vi "Write DIO Threshold.vi"(7 "Logic Threshold (%)":dbl, 8 "error in (no error)":errorcluster, 9 "Chip Address (A2 A1 A0)":T2 max=7, 10 "Slot #":T1 max=15, 11 "Rack #":u8) -> (0 "error out":errorcluster, 3 "FIFO SPI Message":u64 format="%b")   [LabVIEW 2014, in "SLSC configuration Shared.lvlib"]
uses:
  SLSC configuration Shared.lvlib
  MCP23S17/Chip Address.ctl
  SPI Utility/Slot #.ctl
  MCP23S17/IOCON BANK 0 Reg Addresses.ctl
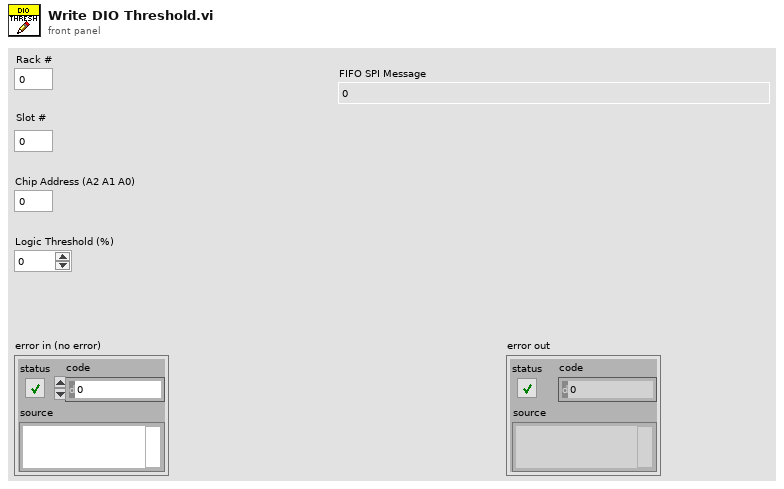
[diagram p1: front panel]
types:
  T1 = typedef "SLSC configuration Shared.lvlib/Slot #.ctl" = u8
  T2 = typedef "SLSC configuration Shared.lvlib/Chip Address.ctl" = u8
  T3 = typedef "SLSC configuration Shared.lvlib/IOCON BANK 0 Reg Addresses.ctl" = enum8{"IODIRA", "IODIRB", "IPOLA", "IPOLB", "GPINTENA", "GPINTENB", "DEFVALA", "DEFVALB", "INTCONA", "INTCONB", "IOCONA", "IOCONB", "GPPUA", "GPPUB", "INTFA", "INTFB", "INTCAPA", "INTCAPB", "GPIOA", "GPIOB", "OLATA", "OLATB"}
  T4 = typedef "SLSC configuration Shared.lvlib/SPI Command.ctl" = cluster{"SPI Command":u32, "Transfer Length":u8}
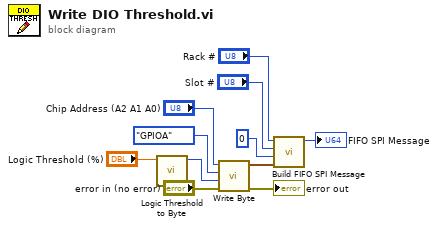
[diagram p0: block diagram]
diagram:
  n1 = call "Logic Threshold to Byte.vi"("Logic Threshold (%)"="Logic Threshold (%)") -> ("Threshold Byte"=w2:u8)  [unwired: 10 in]
  n2 = call "Write Byte.vi"("error in (no error)"="error in (no error)", "Value"=w2, "Reg Address"=IOCON_BANK_0_Reg_Addresses."GPIOA", "Chip Address (A2 A1 A0)"="Chip Address (A2 A1 A0)") -> ("error out"=→"error out":errorcluster, "SPI Command"=w8:T4)  [unwired: 6 in]
  n3 = call "Build FIFO SPI Message.vi"("SPI Command"=w8, "Chip Select"=u8 0, "Slot #"="Slot #", "Rack #"="Rack #") -> ("FIFO SPI Message"=→"FIFO SPI Message":u64)  [unwired: 7 in]
